vi "Run.vi"(8 "error in (no error)":errorcluster caption="entrée d'erreur (pas d'erreur)", 11 "Blobs.lvclass":refnum<class "Blobs.lvclass">) -> (0 "error out":errorcluster caption="sortie d'erreur", 2 "Data":T1, 3 "Blobs.lvclass":refnum<class "Blobs.lvclass">)   [LabVIEW 2020, in "Blobs.lvclass"]
doc: "Returns :\n\nX : array of shape [n_samples, n_features]\n The generated samples.\n\ny : array of shape [n_samples]\n The integer labels for cluster membership of each sample.\n\ncenters : array, shape [n_centers, n_features]\n The centers of each cluster. Only returned if return_centers=True."
uses:
  Blobs.lvclass
  Blobs.lvclass/Blobs.ctl
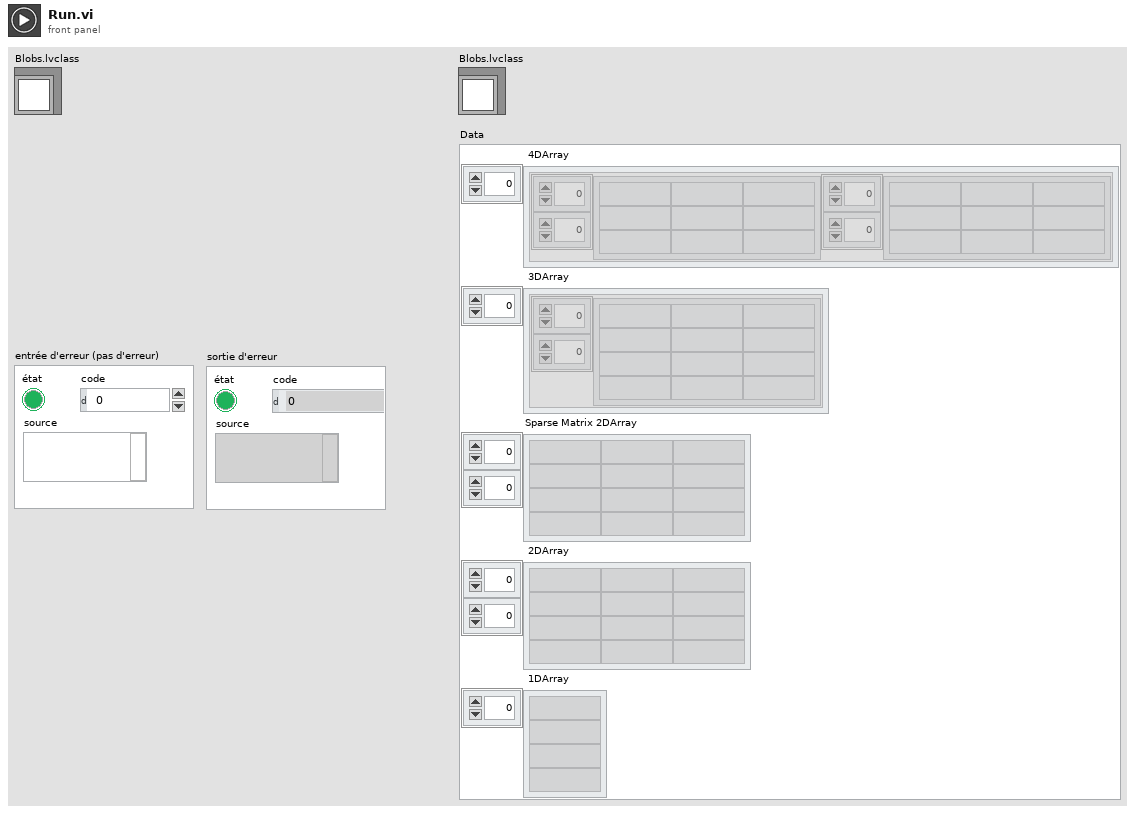
[diagram p1: front panel]
types:
  T1 = cluster{" 4DArray":cluster{"1":string[][], "2":string[][]}[], " 3DArray":cluster{"Tableau":string[][]}[], "Sparse Matrix 2DArray":string[][], " 2DArray":string[][], " 1DArray":string[]}
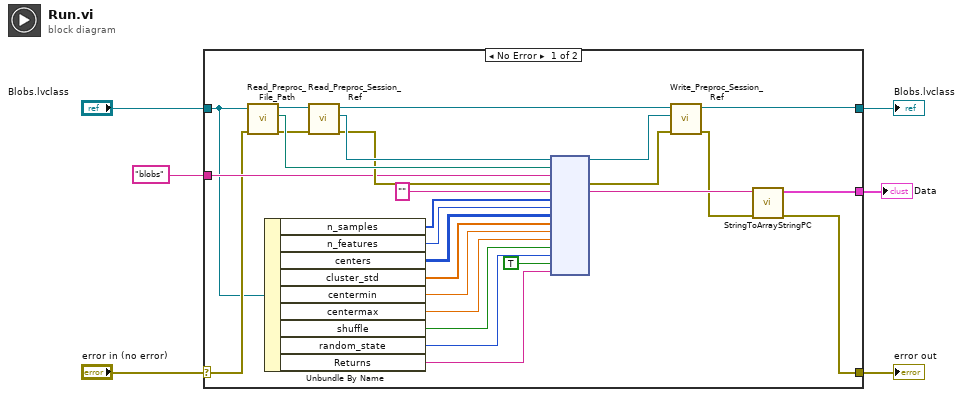
[diagram p0: block diagram]
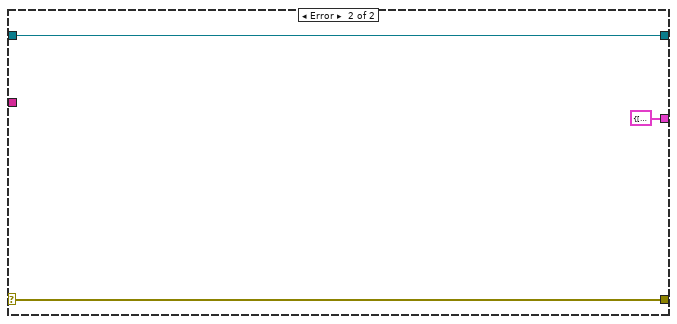
[diagram p2: hidden frame]
diagram:
  n1 = case shown="No Error" "error in (no error)" {
    selector: "error in (no error)" -> [w23 w36]
    tunnel: [w8 w36] -> w5
    tunnel: [w11 w35] -> w3
    tunnel: "Blobs.lvclass" -> [w22 w35]
    tunnel: "blobs" ("Fonction") -> [w24 _]
    tunnel: [w7 T1 {" 4DArray"=[], " 3DArray"=[], "Sparse Matrix 2DArray"=[], " 2DArray"=[], " 1DArray"=[]} ("Data")] -> w1
    frame No Error {
      n2 = call-dynamic "Read_Preproc_File_Path.vi"("error in (no error)"=w23, "Python in"=w22) -> ("error out"=w28:errorcluster, "File_Path"=w31:path, "Python out"=w33:refnum<class "Blobs.lvclass">)  [unwired: 7 in]
      n3 = Unbundle By Name(w22) -> ("n_samples"=w21:i32[], "n_features"=w20:u32, "centers"=w19:i32[][], "cluster_std"=w18:dbl[], "centermin"=w17:dbl, "centermax"=w16:dbl, "shuffle"=w15:bool, "random_state"=w14:i32, "Returns"=w12:string)
      n4 = call-dynamic "Read_Preproc_Session_Ref.vi"("error in (no error)"=w28, "Python in"=w33) -> ("error out"=w29:errorcluster, "Session_ref"=w30:refnum<k35>, "Python out"=w32:refnum<class "Blobs.lvclass">)  [unwired: 7 in]
      n5 = node(w30, w31, w24, w29, "", w21, w20, w19, w18, w17, w16, w15, w14, TRUE, w12) -> (w25:refnum<k35>, w27:errorcluster, w10:string)  [unwired: 10 in, 2 out]
      n6 = call-dynamic "Write_Preproc_Session_Ref.vi"("error in (no error)"=w27, "Session_ref"=w25, "Python in"=w32) -> ("error out"=w9:errorcluster, "Python out"=w11:refnum<class "Blobs.lvclass">)  [unwired: 7 in]
      n7 = call "StringToArrayStringPC.vi"("sortie d'erreur"=w9, "Return value"=w10) -> ("sortie d'erreur"=w8:errorcluster, "Data"=w7:T1)  [unwired: 8 in]
    }
    frame Error {
    }
  }
  "error out" <- w5
  "Blobs.lvclass" <- w3
  "Data" <- w1
